vi "Control_Panel_Test.vi"(11 "Joystick_In":T1) -> ()   [LabVIEW 2019]
uses:
  Globals/Control_Panel_Globals.vi
  Subsystems/Control_Panel/Control_Panel_Cluster.ctl
  Utility_VIs/Joystick_Controls.ctl
panel:
  in  "Control_Panel_Speed":dbl=1.0
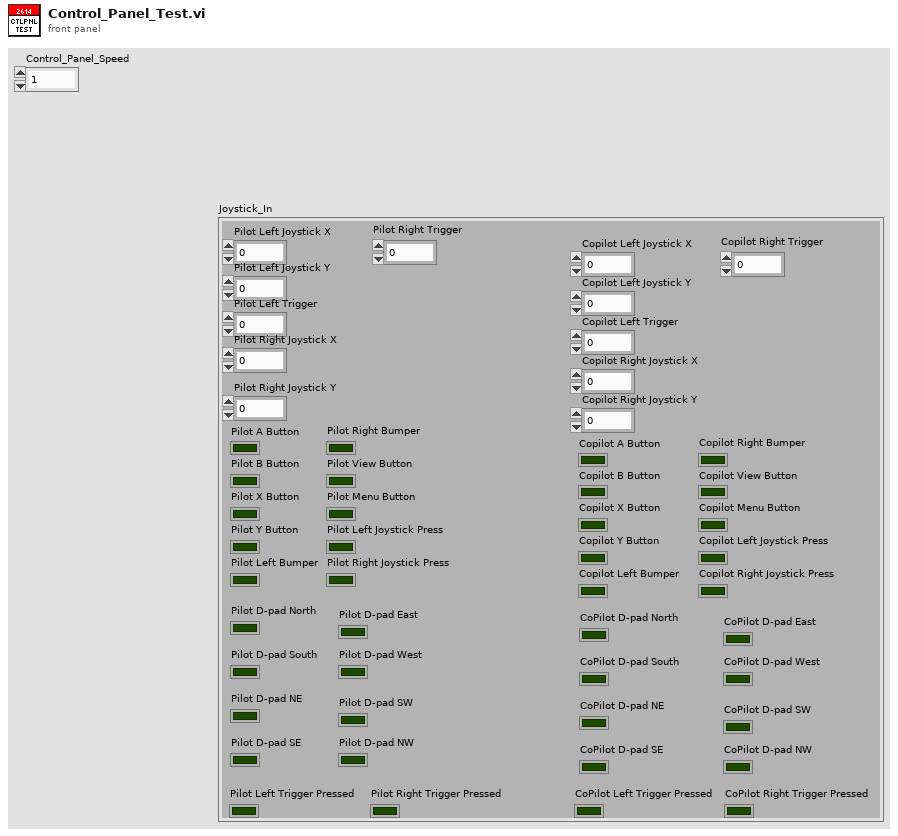
[diagram p1: front panel]
types:
  T1 = typedef "Joystick_Controls.ctl" = cluster{"Pilot Left Joystick X":dbl, "Pilot Left Joystick Y":dbl, "Pilot A Button":bool, "Pilot B Button":bool, "Pilot X Button":bool, "Pilot Y Button":bool, "Pilot Left Bumper":bool, "Pilot Right Bumper":bool, "Pilot View Button":bool, "Pilot Menu Button":bool, "Pilot Left Joystick Press":bool, "Pilot Right Joystick Press":bool, "Pilot Left Trigger":dbl, "Pilot Right Joystick X":dbl, "Pilot Right Joystick Y":dbl, "Pilot Right Trigger":dbl, "Copilot Left Joystick X":dbl, "Copilot Left Joystick Y":dbl, "Copilot A Button":bool, "Copilot B Button":bool, "Copilot X Button":bool, "Copilot Y Button":bool, "Copilot Left Bumper":bool, "Copilot Right Bumper":bool, "Copilot View Button":bool, "Copilot Menu Button":bool, "Copilot Left Joystick Press":bool, "Copilot Right Joystick Press":bool, "Copilot Left Trigger":dbl, "Copilot Right Joystick X":dbl, "Copilot Right Joystick Y":dbl, "Copilot Right Trigger":dbl, "Pilot D-pad North":bool, "Pilot D-pad South":bool, "Pilot D-pad East":bool, "Pilot D-pad West":bool, "Pilot D-pad NE ":bool, "Pilot D-pad SE":bool, "Pilot D-pad SW":bool, "Pilot D-pad NW":bool, "CoPilot D-pad North":bool, "CoPilot D-pad South":bool, "CoPilot D-pad East":bool, "CoPilot D-pad West":bool, "CoPilot D-pad NE":bool, "CoPilot D-pad SE":bool, "CoPilot D-pad SW":bool, "CoPilot D-pad NW":bool, "Pilot Left Trigger Pressed":bool, "Pilot Right Trigger Pressed":bool, "CoPilot Left Trigger Pressed":bool, "CoPilot Right Trigger Pressed":bool}
  T2 = typedef "Control_Panel_Cluster.ctl" = cluster{"Control_State":enum16{"No-Op", "Rotational_Control", "Positional_Control", "Manual_Control"}, "Start_Movement":bool, "Abort":bool, "Rotation_Control?":bool, "Positional_Control? ":bool, "Throttle":dbl}
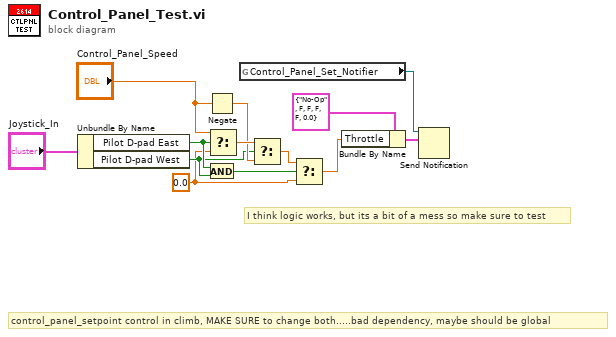
[diagram p0: block diagram]
diagram:
  w1 = 0.0 ("f")
  # "I think logic works, but its a bit of a mess so make sure to test"
  # "control_panel_setpoint control in climb, MAKE SURE to change both.....bad dependency, maybe should be global"
  n1 = Unbundle By Name("Joystick_In") -> ("Pilot D-pad East"=w3:bool, "Pilot D-pad West"=w2:bool)
  n2 = Negate(x="Control_Panel_Speed") -> (-x=w8:dbl)
  n3 = And(x=w3, y=w2) -> (x .and. y?=w4:bool)
  n4 = Select(t="Control_Panel_Speed", s=w3, f=w1) -> (s? t:f=w9:dbl)
  n5 = global read "Control_Panel_Globals.vi" "Control_Panel_Set_Notifier"() -> (w12:refnum<notifier>)
  n6 = Select(t=w9, s=w2, f=w8) -> (s? t:f=w6:dbl)
  n7 = Select(t=w6, s=w4, f=w1) -> (s? t:f=w5:dbl)
  n8 = Bundle By Name(cluster=T2 {"Control_State"=enum."No-Op", "Start_Movement"=FALSE, "Abort"=FALSE, "Rotation_Control?"=FALSE, "Positional_Control? "=FALSE, "Throttle"=0.0} ("notification"), "Throttle"=w5) -> (w10:T2)
  n9 = Send Notification(notification=w10, notifier=w12) -> ()  [unwired: 1 in, 2 out]
